vi "Make String Length Constant.vi"(8 "error in (no error)":errorcluster, 9 "String Lenght":i32=20, 10 "String in":string, 11 "Readout Charact in":refnum<class "Readout Charact.lvclass">) -> (0 "error out":errorcluster, 2 "String out":string, 3 "Readout Charact out":refnum<class "Readout Charact.lvclass">)   [LabVIEW 2018, in "Readout Charact.lvclass"]
uses:
  Readout Charact.lvclass
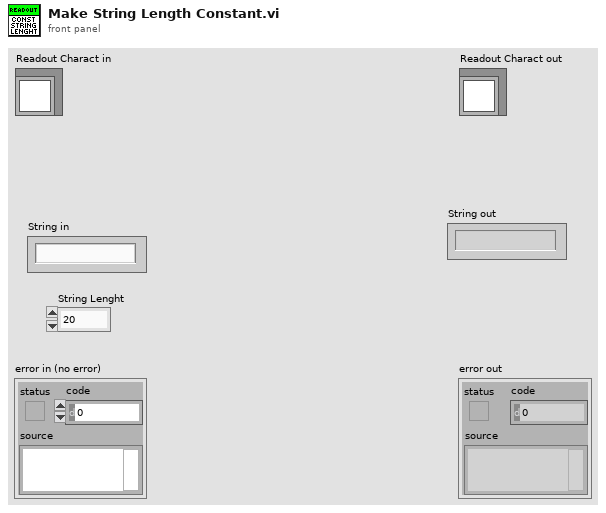
[diagram p1: front panel]
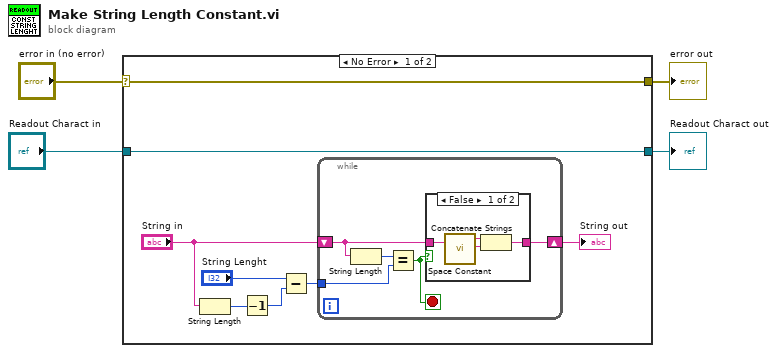
[diagram p0: block diagram]
diagram:
  n1 = case shown="No Error" "error in (no error)" {
    selector: "error in (no error)" -> [w11 w23]
    tunnel: [w11 w23] -> w3
    tunnel: [w12 w22] -> w1
    tunnel: "Readout Charact in" -> [w12 w22]
    frame No Error {
      n2 = String Length(string="String in") -> (length=w8:i32)
      n3 = Decrement(x=w8) -> (x-1=w6:i32)
      n4 = Subtract(x="String Lenght", y=w6) -> (x-y=w5:i32)
      n5 = while {
        tunnel: w5 -> [w16]
        shift-right: [w14] -> w10
        shift-left: "String in" -> [w15]
        stop <- w13 stop-if-true
        n6 = String Length(string=w15) -> (length=w17:i32)
        n7 = Equal?(x=w17, y=w16) -> (x = y?=w13:bool)
        n8 = case shown="False" w13 {
          tunnel: w15 -> [w20 w21]
          tunnel: [w19 w21] -> w14
          frame False {
            n9 = call <vilib>:"Space Constant.vi"() -> ("String"=w18:string)
            n10 = Concatenate Strings(w20, w18) -> (w19:string)
          }
          frame True {
          }
        }
      }
      "String out" <- w10
    }
    frame Error {
    }
  }
  "error out" <- w3
  "Readout Charact out" <- w1
